vi "Cryostation.Get DBL.vi"(8 "error in (no error)":errorcluster, 10 "Command":string, 11 "connection ID in":refnum<k5>) -> (0 "error out":errorcluster, 2 "Response":dbl, 3 "connection ID out":refnum<k5>)   [LabVIEW 2019, in "instrument.Cryostation.lvclass"]
uses:
  instrument.Cryostation.lvclass
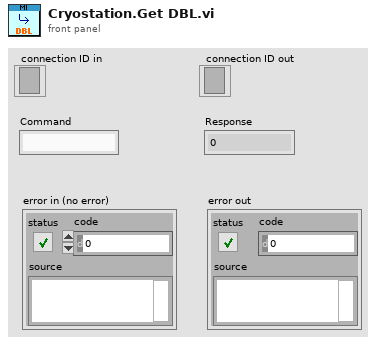
[diagram p1: front panel]
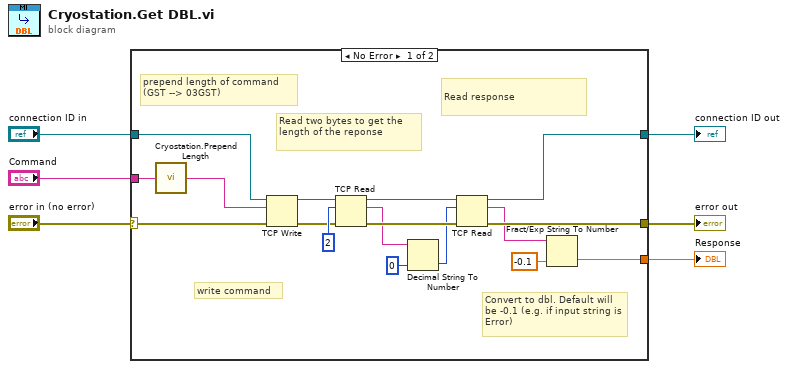
[diagram p0: block diagram]
diagram:
  n1 = case shown="No Error" "error in (no error)" {
    selector: "error in (no error)" -> [w22 w25]
    tunnel: [w8 w24] -> w6
    tunnel: "Command" -> [w11 _]
    tunnel: "connection ID in" -> [w9 w24]
    tunnel: [w23 _] -> w4
    tunnel: [w21 w25] -> w3
    frame No Error {
      # "Convert to dbl. Default will be -0.1 (e.g. if input string is Error)"
      # "Read response"
      # "write command"
      # "Read two bytes to get the length of the reponse"
      # "prepend length of command\n(GST --> 03GST)"
      n2 = call "Cryostation.Prepend Length.vi"("Command"=w11) -> ("0#Command"=w10:string)
      n3 = TCP Write(connection ID=w9, data in=w10, error in (no error)=w22) -> (connection ID out=w19:refnum<k5>, error out=w18:errorcluster)  [unwired: 1 in, 1 out]
      n4 = TCP Read(connection ID=w19, bytes to read=2, error in (no error)=w18) -> (connection ID out=w15:refnum<k5>, data out=w7:string, error out=w14:errorcluster)  [unwired: 2 in]
      n5 = Decimal String To Number(string=w7, default (0L)=0 ("default (0 I32)")) -> (number=w13:i32)  [unwired: 1 in, 1 out]
      n6 = TCP Read(connection ID=w15, bytes to read=w13, error in (no error)=w14) -> (connection ID out=w8:refnum<k5>, data out=w12:string, error out=w21:errorcluster)  [unwired: 2 in]
      n7 = Fract/Exp String To Number(string=w12, default (0 dbl)=-0.1 ("default (0 DBL)")) -> (number=w23:dbl)  [unwired: 2 in, 1 out]
    }
    frame Error {
    }
  }
  "connection ID out" <- w6
  "Response" <- w4
  "error out" <- w3
